vi "Cleanup.vi"(8 "error in (no error)":errorcluster, 11 "CodeCoverage in":refnum<class "CodeCoverage.lvclass">) -> (0 "error out":errorcluster)   [LabVIEW 2019, in "CodeCoverage.lvclass"]
doc: "Stops code coverage measurement and clears the context."
uses:
  CodeCoverage.lvclass
  CodeCoverage.lvclass/CodeCoverage.ctl
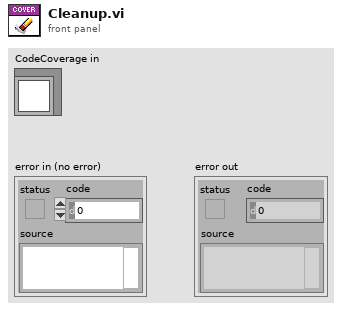
[diagram p1: front panel]
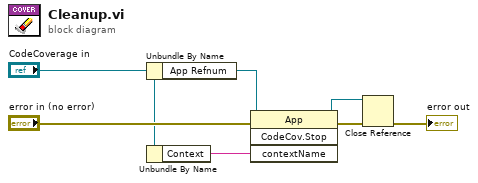
[diagram p0: block diagram]
diagram:
  n1 = Unbundle By Name("CodeCoverage in") -> ("App Refnum"=w2:refnum<vi>)
  n2 = Unbundle By Name("CodeCoverage in") -> ("Context"=w7:string)
  n3 = invoke class="App" method="CodeCov.Stop"(reference=w2, error in="error in (no error)", "contextName"=w7) -> (reference out=w1:refnum<vi>, error out=w3:errorcluster)  [unwired: 1 in, 2 out]
  n4 = Close Reference(reference=w1, error in (no error)=w3) -> (error out=→"error out":errorcluster)
